vi "post-reset-conditional-disable.vi"(5 "Files Generated by Build":path[](array[path]), 6 "Top Level/Always Included VIs":path[](array[path]), 7 "Destination Path":path, 8 "error in (no error)":errorcluster, 9 "Target Name":string, 10 "Build Specification Name":string, 11 "Project Path":path) -> (0 "error out":errorcluster)   [LabVIEW 2019]
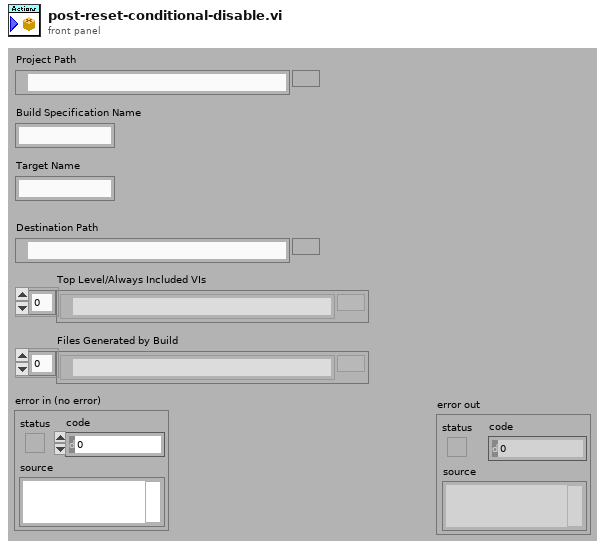
[diagram p1: front panel]
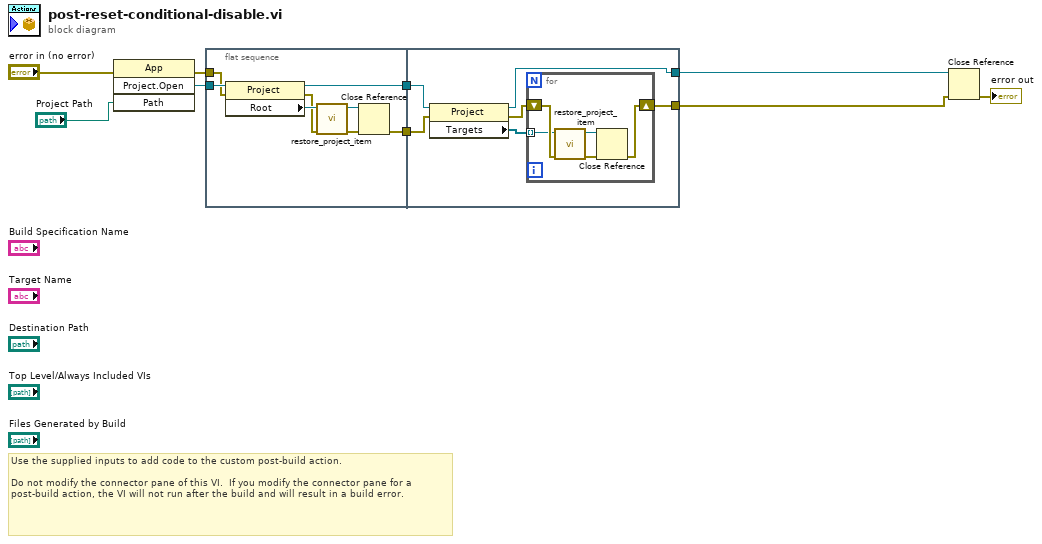
[diagram p0: block diagram]
diagram:
  # "Use the supplied inputs to add code to the custom post-build action.\n\nDo not modify the connector pane of this VI.  If you modify the connector pane for a post-build action, the VI will not run after the build and will result in a build error."
  n1 = invoke class="App" method="Project.Open"(error in="error in (no error)", "Path"="Project Path") -> (error out=w7:errorcluster, "Project:Open"=w9:refnum<vi>)  [unwired: 2 in, 2 out]
  n2 = flat-sequence {
    tunnel: w9 -> [w17]
    tunnel: w7 -> [w13]
    tunnel: [w11] -> w2
    tunnel: [w10] -> w1
    tunnel: [w21] -> w4
    tunnel: [w20] -> w3
    tunnel: w2 -> [w19]
    tunnel: w1 -> [w18]
    frame #0 {
      n3 = property class="Project"(reference=w17, error in=w13) -> (reference out=w10:refnum<vi>, error out=w12:errorcluster, "Root"=w14:refnum<vi>)
      n4 = call "restore_project_item.vi"("error in (no error)"=w12, "ProjectItem in"=w14) -> ("error out"=w16:errorcluster, "ProjectItem out"=w15:refnum<vi>)  [unwired: 8 in]
      n5 = Close Reference(reference=w15, error in (no error)=w16) -> (error out=w11:errorcluster)
    }
    frame #1 {
      n6 = property class="Project"(reference=w18, error in=w19) -> (reference out=w20:refnum<vi>, error out=w23:errorcluster, "Targets"=w22:refnum<vi>[])
      n7 = for {
        tunnel: w22 -> [w27] mode=indexing
        shift-right: [w24] -> w21
        shift-left: w23 -> [w28]
        n8 = call "restore_project_item.vi"("error in (no error)"=w28, "ProjectItem in"=w27) -> ("error out"=w25:errorcluster, "ProjectItem out"=w26:refnum<vi>)  [unwired: 8 in]
        n9 = Close Reference(reference=w26, error in (no error)=w25) -> (error out=w24:errorcluster)
      }
    }
  }
  n10 = Close Reference(reference=w3, error in (no error)=w4) -> (error out=→"error out":errorcluster)
